vi "Master.vi"() -> ()   [LabVIEW 2014]
uses:
  <vilib>/lvdsc/process/Deploy Library.vi
  <vilib>/lvdsc/process/Undeploy Library.vi
  <vilib>/lvdsc/NI_DSC.lvlib
panel:
  out "Error Out":errorcluster
  in  "stop":bool
  out "000005":bool
  out "000004":bool
  out "000003":bool
  out "000002":bool
  out "000001":bool
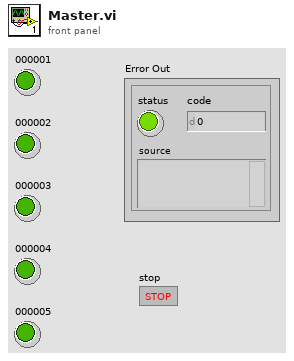
[diagram p1: front panel]
types:
  T1 = cluster{"Read Access":enum8{"Allowed", "Required", "None"}, "Write Access":enum8{"Allowed", "Required", "None"}}
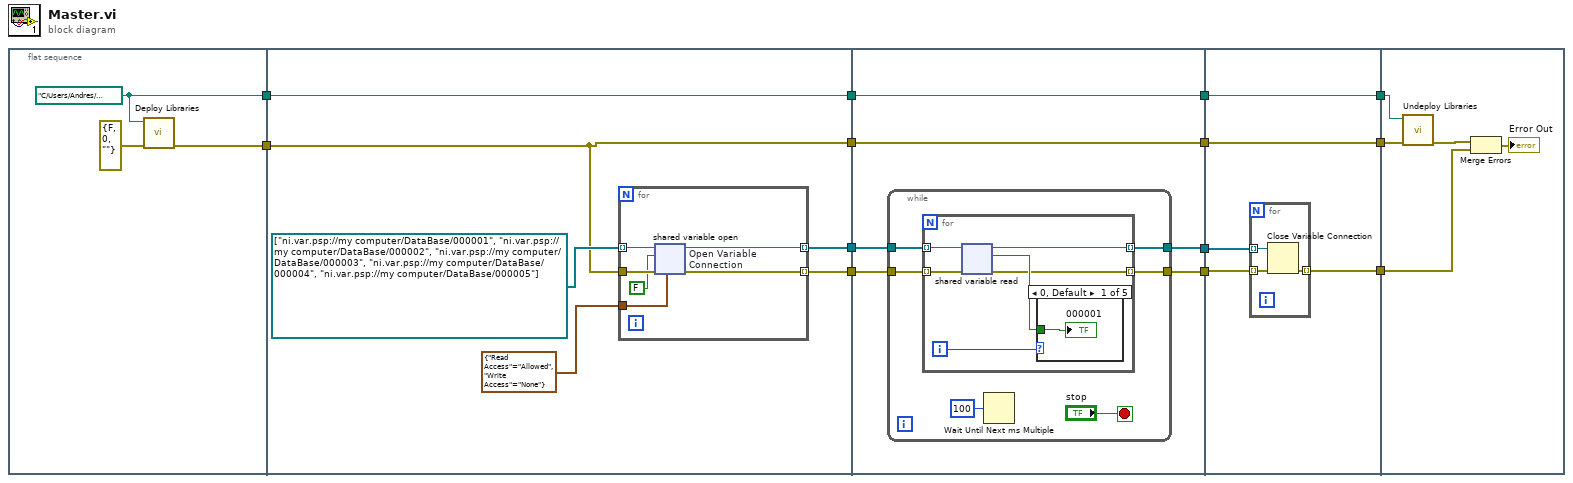
[diagram p0: block diagram]
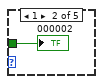
[diagram p2: hidden frame]
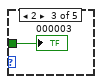
[diagram p3: hidden frame]
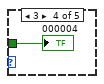
[diagram p4: hidden frame]
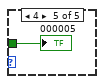
[diagram p5: hidden frame]
diagram:
  n1 = flat-sequence {
    tunnel: [w15] -> w13
    tunnel: [w14] -> w12
    tunnel: w13 -> [w17]
    tunnel: w12 -> [w18]
    tunnel: [w20] -> w11
    tunnel: [w19] -> w10
    tunnel: [w18] -> w4
    tunnel: [w17] -> w1
    tunnel: w11 -> [w34]
    tunnel: w10 -> [w33]
    tunnel: [w32] -> w9
    tunnel: [w31] -> w8
    tunnel: [w30] -> w5
    tunnel: w4 -> [w30]
    tunnel: [w29] -> w2
    tunnel: w1 -> [w29]
    tunnel: w9 -> [w56]
    tunnel: w8 -> [w55]
    tunnel: [w54] -> w7
    tunnel: [w53] -> w6
    tunnel: w5 -> [w53]
    tunnel: [w52] -> w3
    tunnel: w2 -> [w52]
    tunnel: w7 -> [w62]
    tunnel: w6 -> [w61]
    tunnel: w3 -> [w60]
    frame #0 {
      w14 = path "C:/Users/Andres/Documents/MedidorInteligente/Comunicacion/DataBase.lvlib" ("library path")
      n2 = call-poly <vilib>:"Deploy Libraries.vi"("error in (no error)"=errorcluster {"status"=FALSE, "code"=0, "source"=""}, "library path"=w14) -> ("error out"=w15:errorcluster)  [unwired: 7 in]
    }
    frame #1 {
      n3 = for {
        tunnel: w17 -> [w28]
        tunnel: refnum<k21>[] ["ni.var.psp://my computer/DataBase/000001", "ni.var.psp://my computer/DataBase/000002", "ni.var.psp://my computer/DataBase/000003", "ni.var.psp://my computer/DataBase/000004", "ni.var.psp://my computer/DataBase/000005"] -> [w26] mode=indexing
        tunnel: [w25] -> w19 mode=indexing
        tunnel: [w24] -> w20 mode=indexing
        tunnel: T1 {"Read Access"=enum."Allowed", "Write Access"=enum."None"} ("access") -> [w23]
        n4 = shared-variable-open "Open Variable Connection"(w26, w28, FALSE ("data type"), w23) -> (w24:refnum<k21>, w25:errorcluster)
      }
    }
    frame #2 {
      n5 = while {
        tunnel: w34 -> [w40]
        tunnel: w33 -> [w39]
        tunnel: [w36] -> w32
        tunnel: [w35] -> w31
        stop <- "stop" stop-if-true
        n6 = for {
          tunnel: w40 -> [w46] mode=indexing
          tunnel: w39 -> [w45] mode=indexing
          tunnel: [w42] -> w36 mode=indexing
          tunnel: [w41] -> w35 mode=indexing
          i -> [w43]
          n7 = shared-variable-read(w46, w45) -> (w42:refnum<k21>, w41:errorcluster, w44:bool)  [unwired: 1 out]
          n8 = case shown="0, Default" w43 {
            tunnel: w44 -> [w47 w48 w49 w50 w51]
            frame 0, Default {
              "000001" <- w47
            }
            frame 1 {
              "000002" <- w48
            }
            frame 2 {
              "000003" <- w49
            }
            frame 3 {
              "000004" <- w50
            }
            frame 4 {
              "000005" <- w51
            }
          }
        }
        n9 = Wait Until Next ms Multiple(millisecond multiple=u32 100) -> ()  [unwired: 1 out]
      }
    }
    frame #3 {
      n10 = for {
        tunnel: w56 -> [w59] mode=indexing
        tunnel: w55 -> [w58] mode=indexing
        tunnel: [w57] -> w54 mode=indexing
        n11 = Close Variable Connection(8:w58, 11:w59) -> (0:w57:errorcluster)
      }
    }
    frame #4 {
      n12 = call-poly <vilib>:"Undeploy Libraries.vi"("error in (no error)"=w60, "library path"=w61) -> ("error out"=w64:errorcluster)  [unwired: 7 in]
      n13 = Merge Errors(w64, w62) -> (→"Error Out":errorcluster)
    }
  }
